vi "define.vi"(8 "error in (no error)":errorcluster, 11 "TrajectoryMH100122AODRAPS in":refnum<class "TrajectoryMH100122AODRAPS.lvclass">) -> (0 "error out":errorcluster, 3 "TrajectoryMH100122AODRAPS out":refnum<class "TrajectoryMH100122AODRAPS.lvclass">)   [LabVIEW 2010, in "TrajectoryMH100122AODRAPS.lvclass"]
doc: "modal dialog on which the user can set the trajectory parameters"
uses:
  TrajectoryMH100122AODRAPS.lvclass
  common/xcontrols/XImage/XImage/XImage.xctl
  common/classes/ImageCollection/ImageCollection/ImageCollection.lvclass
  roi_visualization_cluster.ctl
  common/xcontrols/XImage/XImage/ROI_mode_enum.ctl
  TrajectoryMH100122AODRAPS.lvclass/TrajectoryMH100122AODRAPS.ctl
  <vilib>/Utility/miscctls.llb/LVPointTypeDef.ctl
  common/classes/SpaceVector/SpaceVector/SpaceVector.lvclass
  class_data.vi
  common/classes/ErrorController/ErrorController/class_data.vi
  common/classes/ErrorController/ErrorController/ErrorController.lvclass
  common/classes/Box/Box/Box.lvclass
panel:
  in  "button: ok":bool
  in  "button: cancel":bool
  in  "button: reset":bool
  in  "XImage":refnum<class "ImageCollection.lvclass">(xcontrol)
  in  "accept switch":bool=TRUE
  in  "reset switch":bool
  in  "cancel switch":bool=TRUE
  in  "tab":enum32{"User", "ROI points", "About"}(tab)
  out "FOVy":dbl[unit]=0.0003
  out "FOVx":dbl[unit]=0.0003
  in  "enable sub-pattern":bool
  in  "enable ROI numbering":bool caption="enable numbering"
  in  "ROI color":u32(colorbox)=4456192 caption="color"
  in  "extrapolate distance":dbl[unit] min=0.0
  in  "z-step size / frame":u16
  in  "z-offset":u16
  out "# points":i32
  out "# ROIs":i32
  in  "# iteration points":dbl
  in  "winding number":dbl=1.0 min=1.0
  in  "height":dbl=1.0 min=1.0
  in  "diameter":dbl[unit]
  in  "button:plot_3d":bool
  in  "roi table out":T1[](array[typedef]) {"type" items=["point", "line", "poly line", "free line"]}
  # "ROIs"
  # "z-stepping"
  # "TrajectoryAODRAPS"
  # "Developed by Marcel van 't Hoff, University of Zurich, Switzerland"
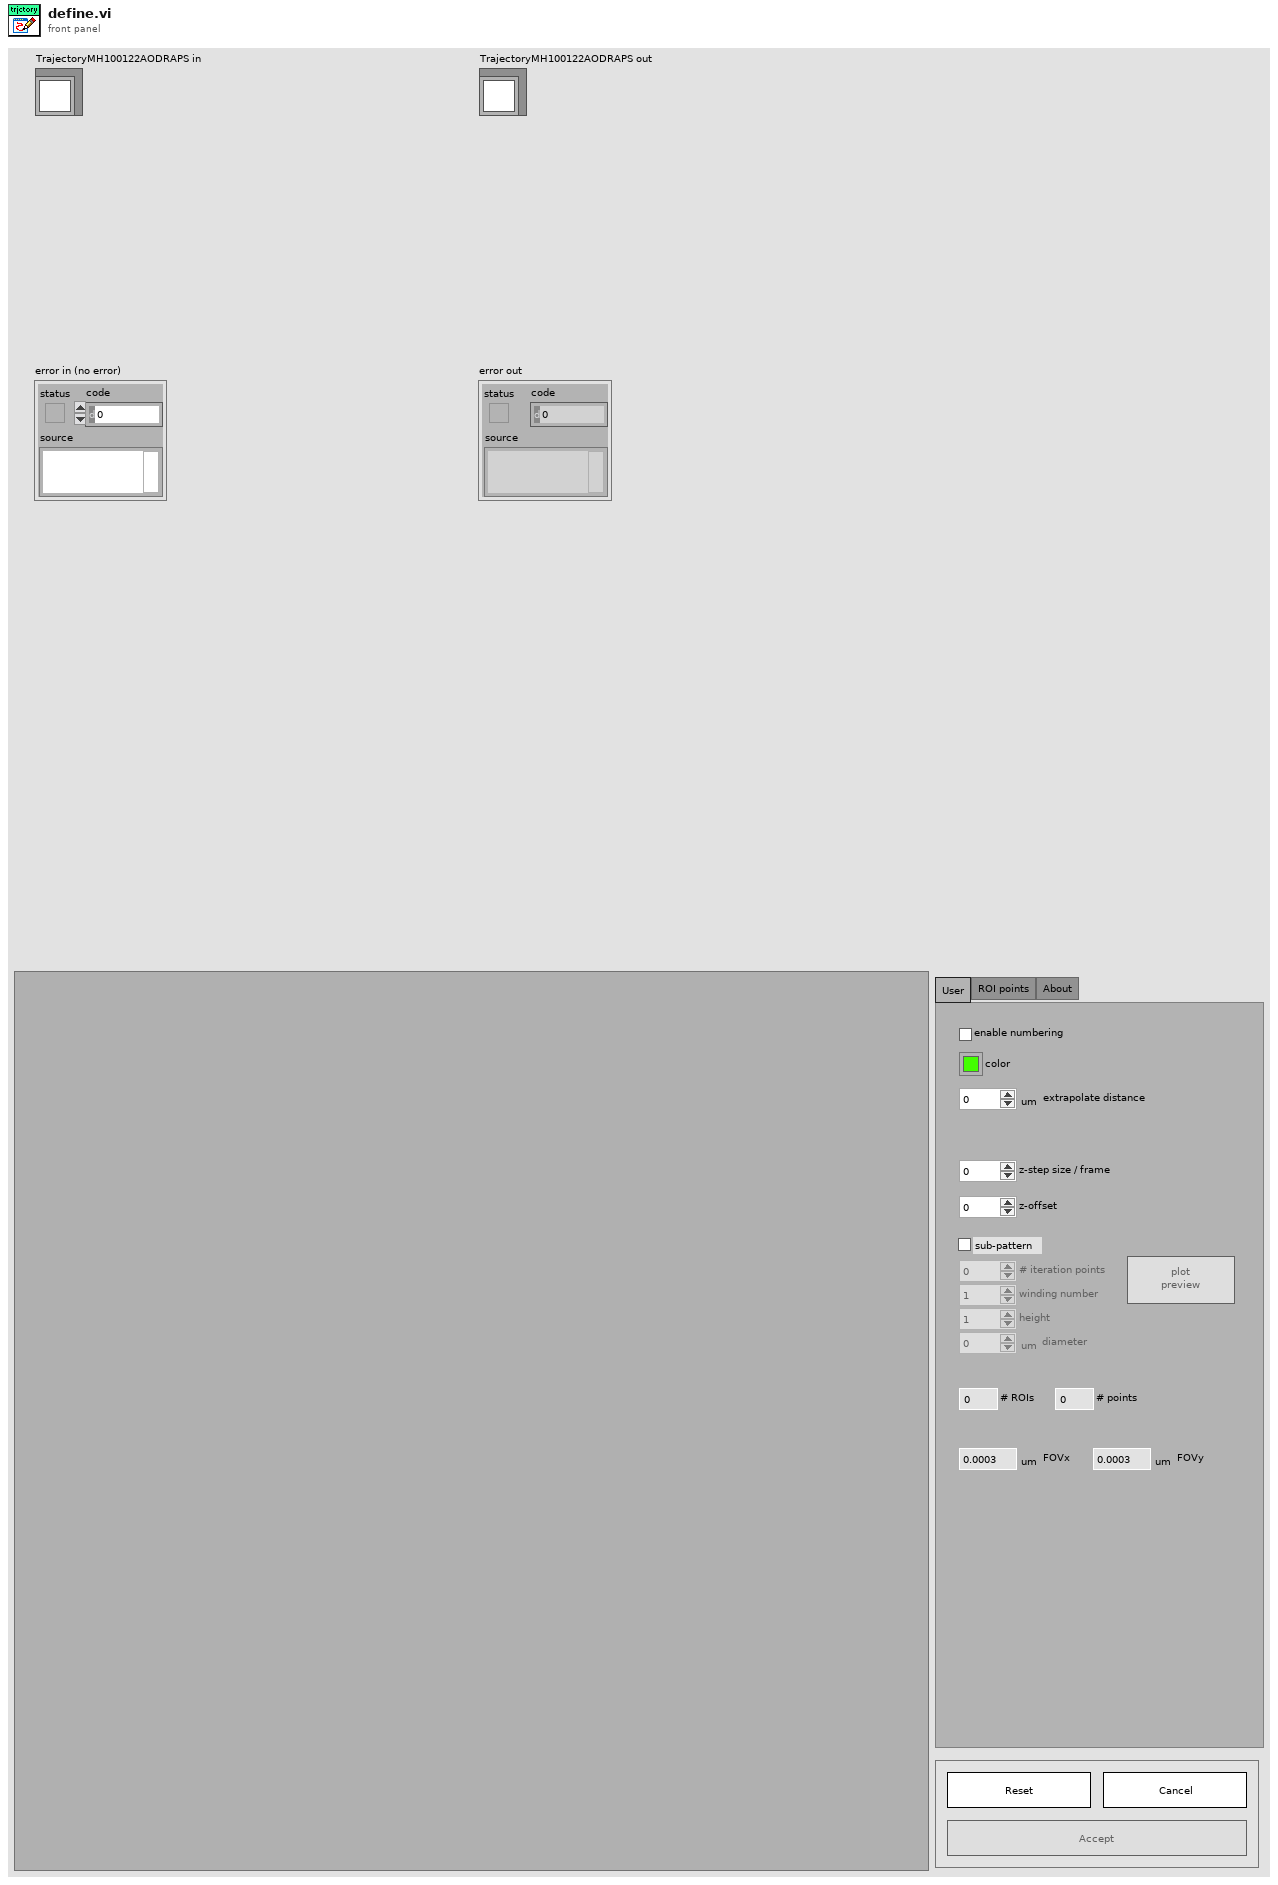
[diagram p1: front panel]
types:
  T1 = typedef "TrajectoryMH100122AODRAPS.lvclass/roi_visualization_cluster.ctl" = cluster{"counter":i32, "type":u16, "activation":enum16{"standard sub-pattern", "long activation"}}
  T2 = typedef "XImage.xctl/ROI_mode_enum.ctl" = enum16{"none", "IMAQROIs", "PointCollection"}
  T3 = typedef "LVPointTypeDef.ctl" = cluster{"Horizontal":i16, "Vertical":i16}
  T4 = cluster{"Global Rectangle":i32[], "Contours":cluster{"Contour Type":u32, "ROI Type":u32, "Points":i32[]}[]}[]
  T5 = enum8{"Enabled", "Disabled", "Disabled and Grayed Out"}
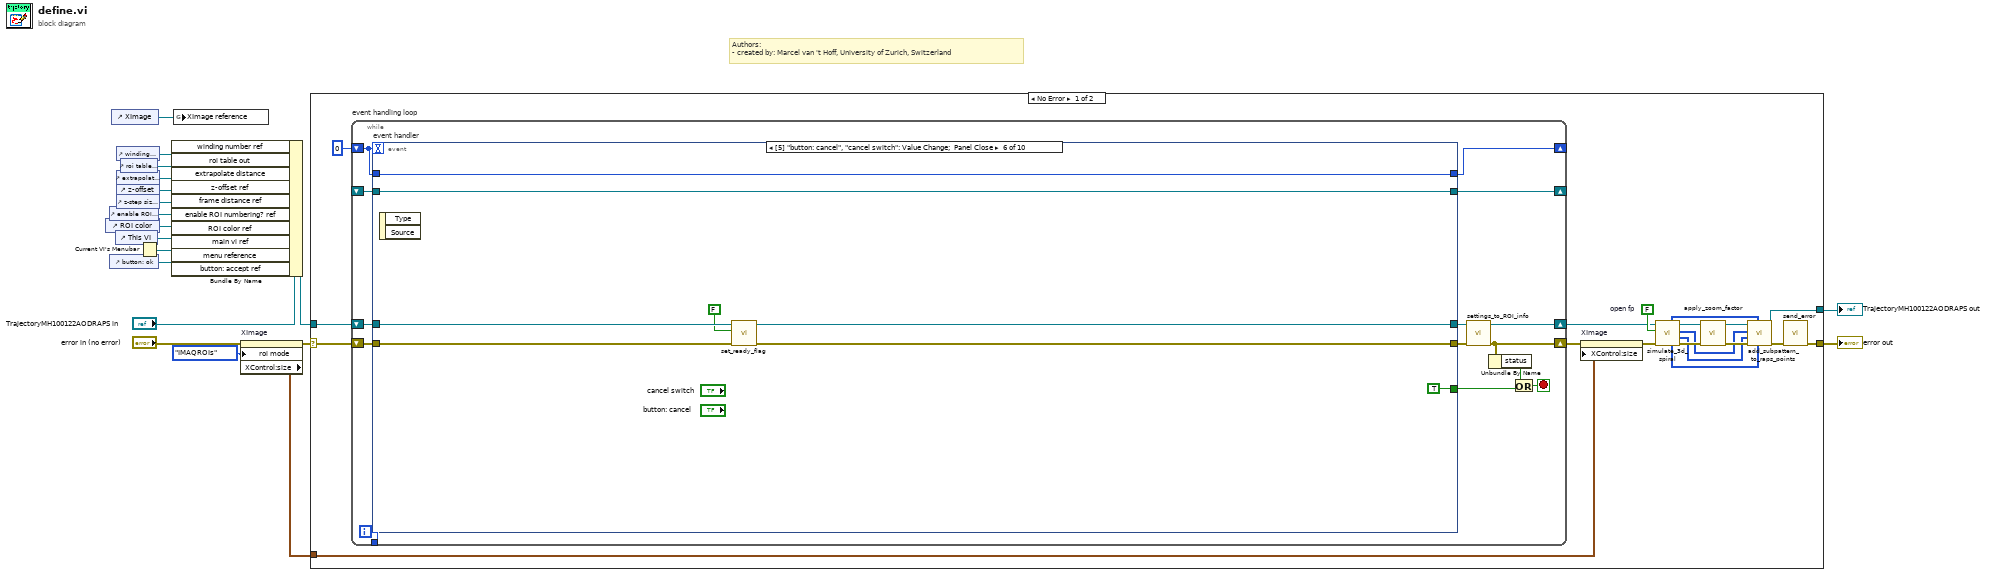
[diagram p0: block diagram]
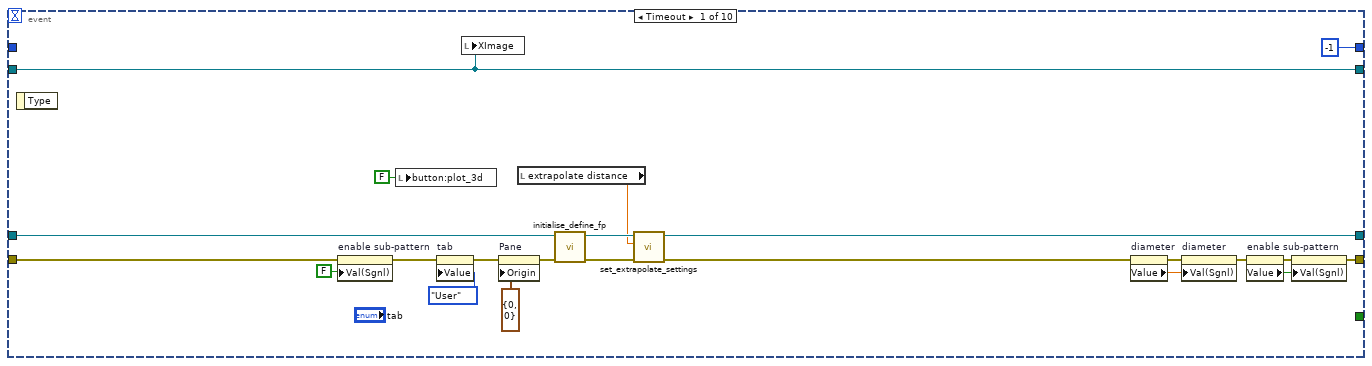
[diagram p2: hidden frame]
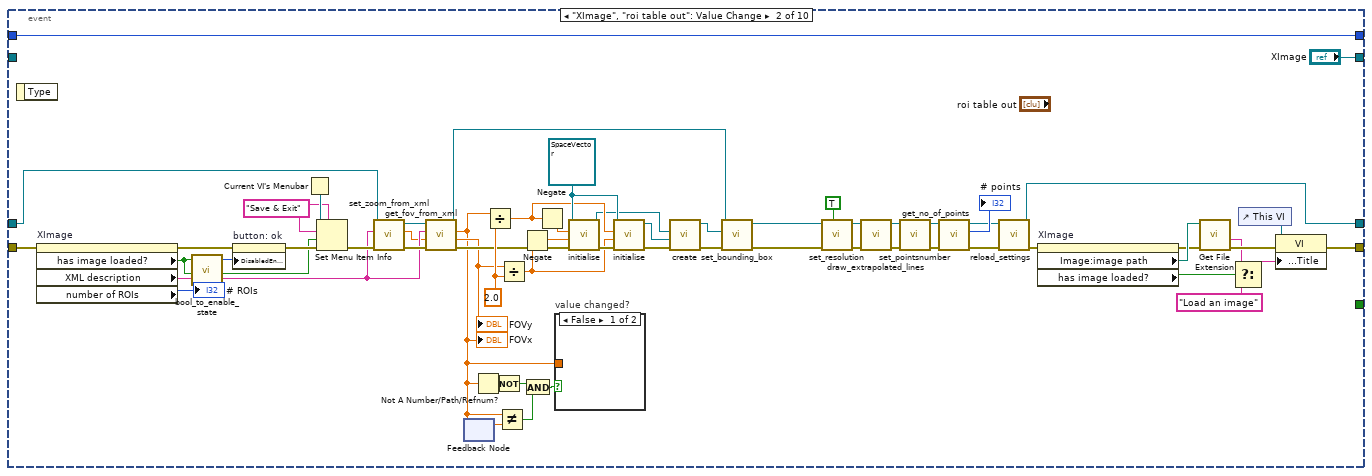
[diagram p3: hidden frame]
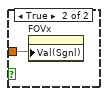
[diagram p4: hidden frame]
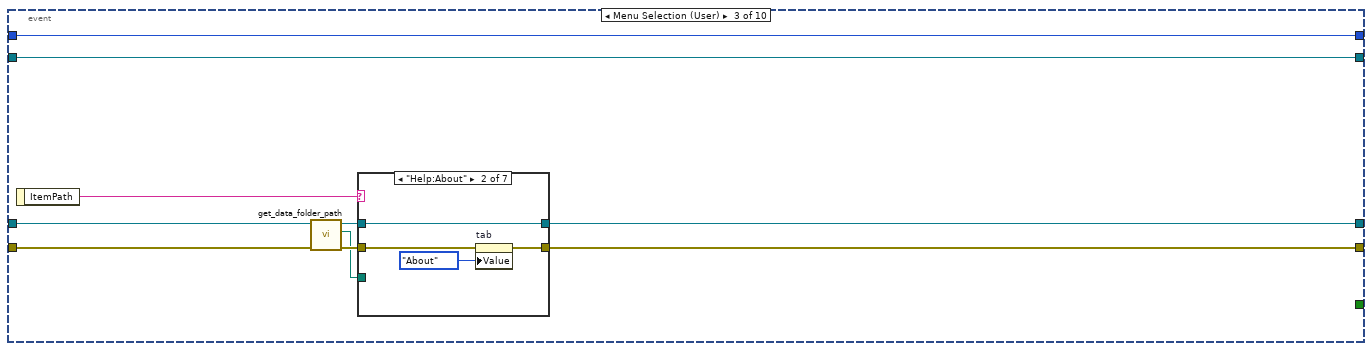
[diagram p5: hidden frame]
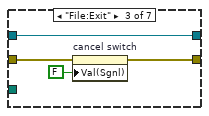
[diagram p7: hidden frame]
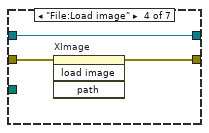
[diagram p8: hidden frame]
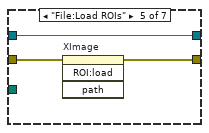
[diagram p9: hidden frame]
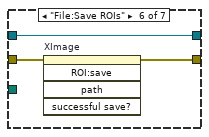
[diagram p10: hidden frame]
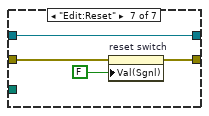
[diagram p11: hidden frame]
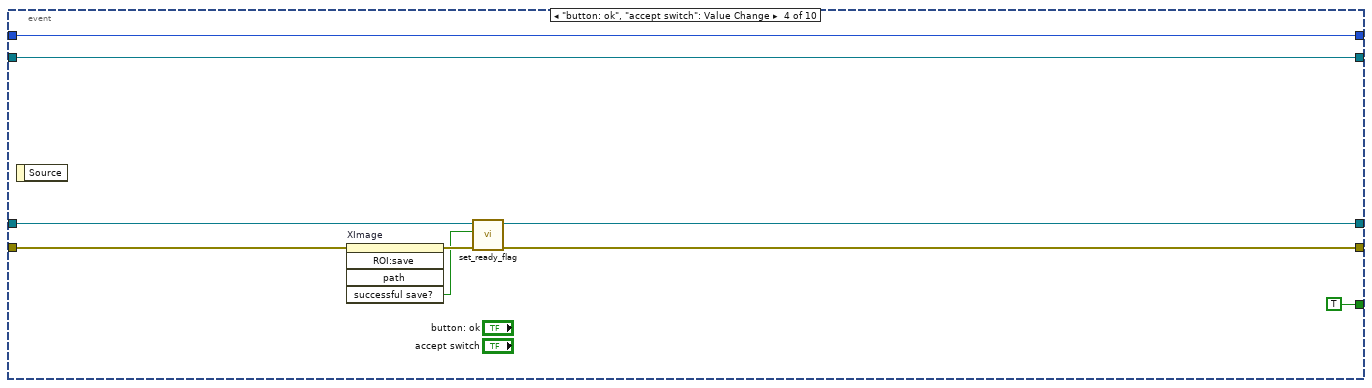
[diagram p12: hidden frame]
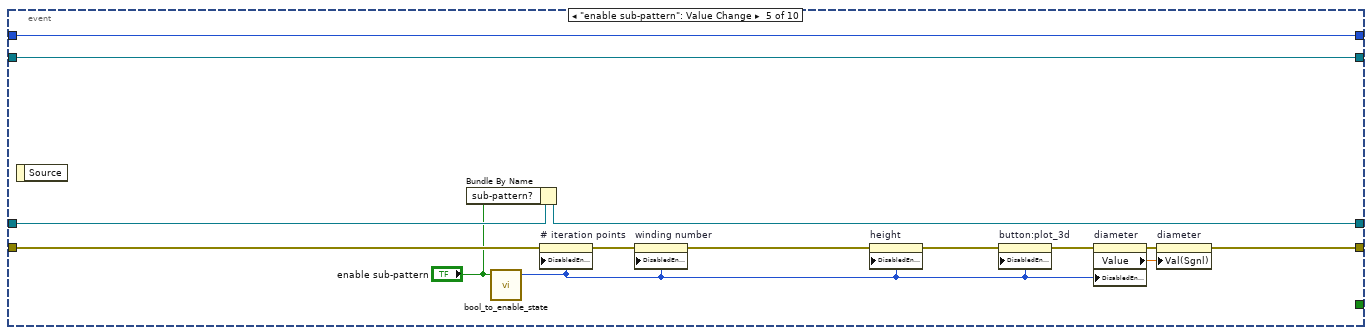
[diagram p13: hidden frame]
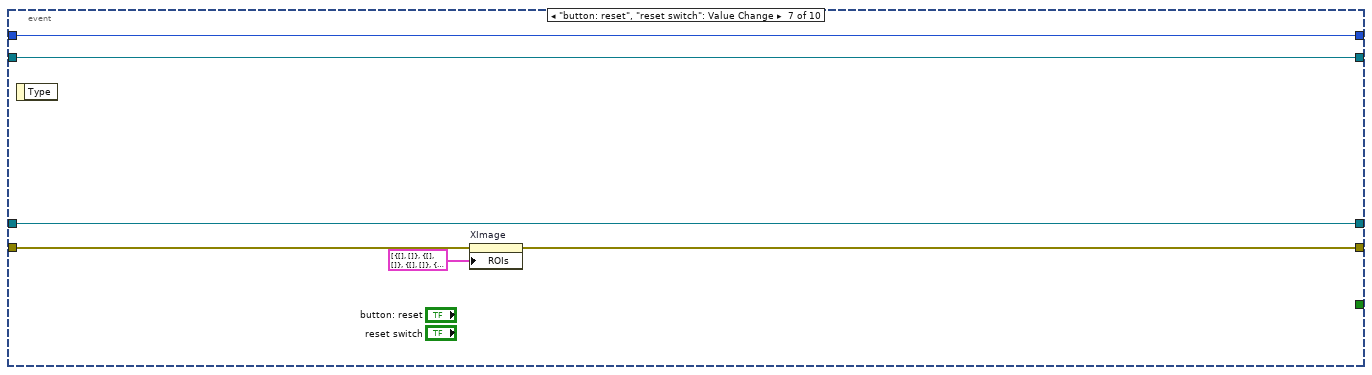
[diagram p14: hidden frame]
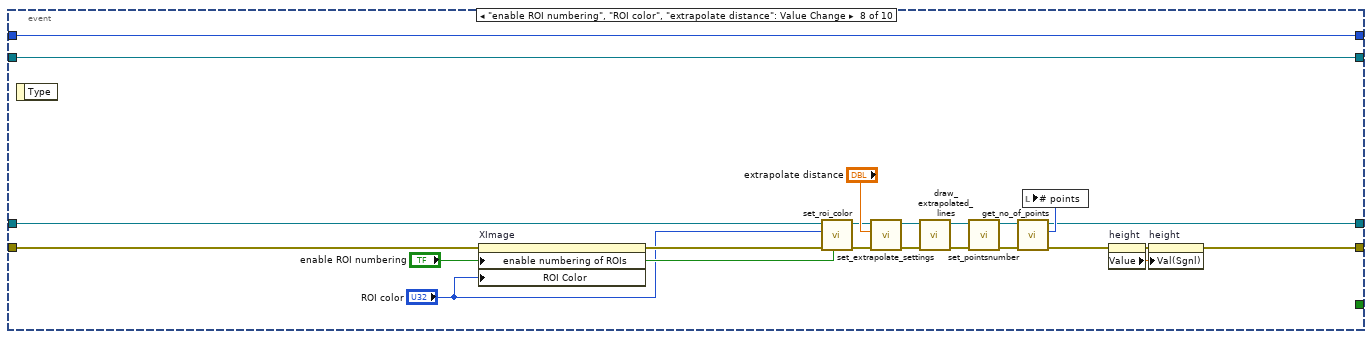
[diagram p15: hidden frame]
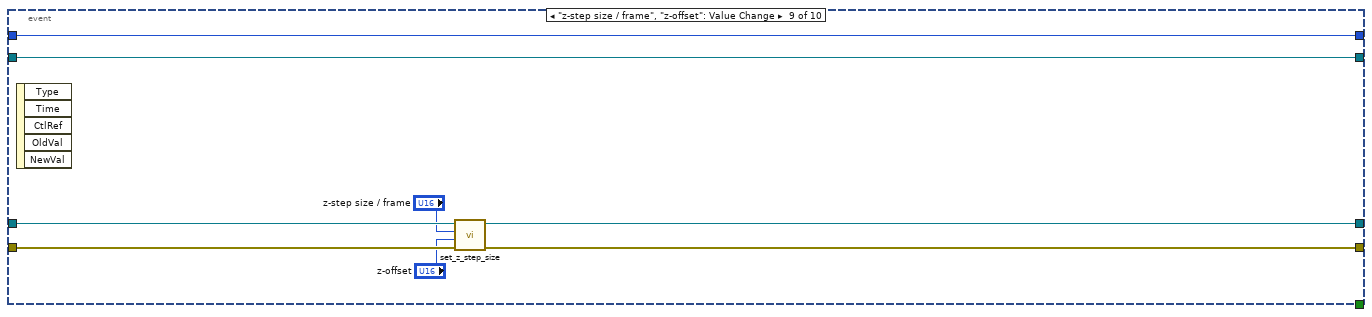
[diagram p16: hidden frame]
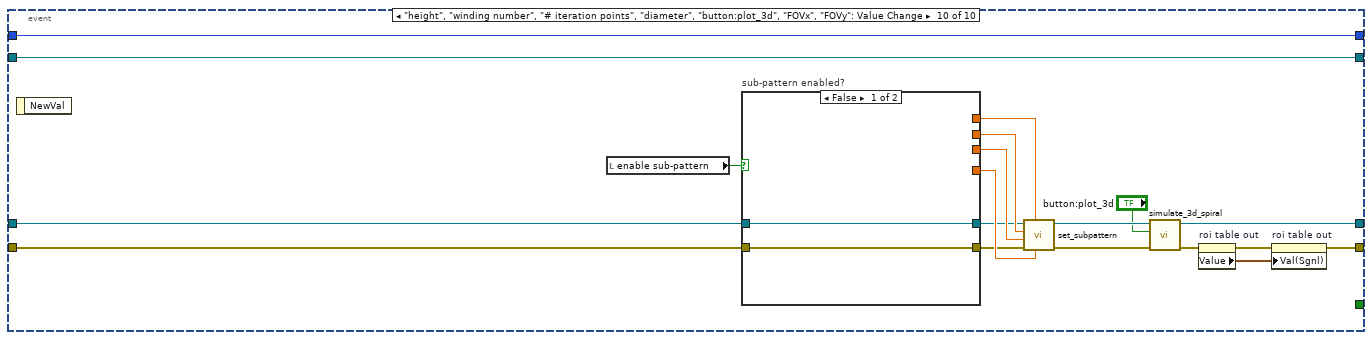
[diagram p17: hidden frame]
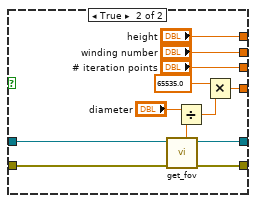
[diagram p18: hidden frame]
diagram:
  # "Authors: \n- created by: Marcel van 't Hoff, University of Zurich, Switzerland"
  n1 = control-ref of="ROI color"() -> (w15:refnum<vi>)
  n2 = control-ref of="enable ROI numbering"() -> (w16:refnum<vi>)
  n3 = control-ref of="button: ok"() -> (w14:refnum<vi>)
  n4 = control-ref of="XImage"() -> (w3:refnum<vi>)
  n5 = control-ref of="This VI"() -> (w12:refnum<vi>)
  n6 = control-ref of="winding number"() -> (w4:refnum<vi>)
  n7 = control-ref of="extrapolate distance"() -> (w8:refnum<vi>)
  n8 = control-ref of="z-offset"() -> (w9:refnum<vi>)
  n9 = control-ref of="z-step size / frame"() -> (w17:refnum<vi>)
  n10 = control-ref of="roi table out"() -> (w5:refnum<vi>)
  n11 = Current VI's Menubar() -> (w13:refnum<k9>)
  n12 = Bundle By Name(cluster="TrajectoryMH100122AODRAPS in", "winding number ref"=w4, "roi table out"=w5, "extrapolate distance"=w8, "z-offset ref"=w9, "frame distance ref"=w17, "enable ROI numbering? ref"=w16, "ROI color ref"=w15, "main vi ref"=w12, "menu reference"=w13, "button: accept ref"=w14) -> (w10:refnum<class "TrajectoryMH100122AODRAPS.lvclass">)
  n13 = global write "class_data.vi" "XImage reference"(w3) -> ()
  n14 = property on="XImage" class="XImage (strict)"(error in="error in (no error)", "roi mode"=ROI_mode_enum."IMAQROIs" ("ROI:mode")) -> (error out=w6:errorcluster, "XControl:size"=w1:cluster{"Width":u32, "Height":u32})  [unwired: 1 in, 1 out]
  n15 = case shown="No Error" w6 {
    selector: w6 -> [w38 w270]
    tunnel: [w35 w270] -> w19
    tunnel: [w24 w269] -> w18
    tunnel: w10 -> [w37 w269]
    tunnel: w1 -> [w33 _]
    frame No Error {
      w32 = FALSE  # open fp
      n16 = while "event handling loop" {
        shift-right: [w43] -> w34
        shift-left: w38 -> [w52]
        shift-right: [w41] -> w30
        shift-left: w37 -> [w49]
        shift-right: [w50] -> _
        shift-left: 0 -> [w51]
        shift-right: [w45] -> _
        shift-left: _ -> [w44]
        tunnel: [w39] -> _
        i -> [w39]
        stop <- w47 stop-if-true
        n17 = event "event handler" shown="[5] \"button: cancel\", \"cancel switch\": Value Change;  Panel Close" {
          selector: _ -> [_ _ _ _ _ _ _ _ _ _]
          dyn-events: _ -> [_ _ _ _ _ _ _ _ _ _]
          timeout: w51 -> [_ _ _ _ _ _ _ _ _ _]
          tunnel: [w55 w111 w143 w175 w178 w197 w203 w206 w232 w240] -> w42
          tunnel: w52 -> [w63 w98 w139 w174 w187 w198 w204 w219 w233 w237]
          tunnel: w51 -> [_ w134 w145 w177 w191 w199 w205 w227 w235 w254]
          tunnel: [-1 w134 w145 w177 w191 w199 w205 w227 w235 w254] -> w50
          tunnel: w49 -> [w66 w99 w141 w176 w185 w196 w202 w225 w231 w236]
          tunnel: [w54 w114 w142 w169 w184 w195 w202 w210 w229 w244] -> w40
          tunnel: [_ _ _ TRUE ("x .or. y?") _ TRUE ("x .or. y?") _ _ _ _] -> w46
          tunnel: [w71 "XImage" w136 w170 w190 w192 w200 w226 w234 w253] -> w45
          tunnel: w44 -> [w71 _ w136 w170 w190 w192 w200 w226 w234 w253]
          event Timeout {
            n18 = event-data() -> ()  [unwired: 1 in, 1 out]
            n19 = property on="enable sub-pattern" class="Bool (strict)"(error in=w63, "Val(Sgnl)"=FALSE ("Value (Signaling)")) -> (error out=w62:errorcluster)  [unwired: 1 in, 1 out]
            n20 = local write "button:plot_3d"(FALSE ("button:plot_3d")) -> ()
            n21 = property on="tab" class="TabCtl (strict)"(error in=w62, "Value"=enum32{"User", "ROI points", "About"}."User" ("tab")) -> (error out=w67:errorcluster)  [unwired: 1 in, 1 out]
            n22 = local write "XImage"(w71) -> ()
            n23 = property on="Pane" class="Pane"(error in=w67, "Origin"=T3 {"Horizontal"=0, "Vertical"=0}) -> (error out=w72:errorcluster)  [unwired: 1 in, 1 out]
            n24 = local read "extrapolate distance"() -> (w68:dbl[unit])
            n25 = call-dynamic "initialise_define_fp.vi"("error in (no error)"=w72, "TrajectoryMH100122AODRAPS in"=w66) -> ("error out"=w69:errorcluster, "TrajectoryMH100122AODRAPS out"=w70:refnum<class "TrajectoryMH100122AODRAPS.lvclass">)  [unwired: 8 in]
            n26 = call-dynamic "set_extrapolate_settings.vi"("error in (no error)"=w69, "extrapolate distance"=w68, "TrajectoryMH100122AODRAPS in"=w70) -> ("error out"=w53:errorcluster, "TrajectoryMH100122AODRAPS out"=w54:refnum<class "TrajectoryMH100122AODRAPS.lvclass">)  [unwired: 7 in]
            n27 = property on="diameter" class="DigNum (strict)"(error in=w53) -> (error out=w59:errorcluster, "Value"=w60:dbl[unit])  [unwired: 1 in, 1 out]
            n28 = property on="diameter" class="DigNum (strict)"(error in=w59, "Val(Sgnl)"=w60) -> (error out=w56:errorcluster)  [unwired: 1 in, 1 out]
            n29 = property on="enable sub-pattern" class="Bool (strict)"(error in=w56) -> (error out=w57:errorcluster, "Value"=w58:bool)  [unwired: 1 in, 1 out]
            n30 = property on="enable sub-pattern" class="Bool (strict)"(error in=w57, "Val(Sgnl)"=w58) -> (error out=w55:errorcluster)  [unwired: 1 in, 1 out]
          }
          event "XImage", "roi table out": Value Change {
            w96 = refnum<class "SpaceVector.lvclass"> refnum ("SpaceVector in")
            w97 = 2.0
            w126 = "Save & Exit" ("item tag")
            n31 = event-data() -> ()  [unwired: 1 in, 1 out]
            n32 = property on="XImage" class="XImage (strict)"(error in=w98) -> (error out=w133:errorcluster, "has image loaded?"=w127:bool, "XML description"=w100:string, "number of ROIs"=→"# ROIs":i32)  [unwired: 1 in, 1 out]
            n33 = call "bool_to_enable_state.vi"("boolean in"=w127) -> ("enabled status out"=w132:T5)  [unwired: 4 in]
            n34 = property on="button: ok" class="Bool"(error in=w133, "DisabledEnum"=w132) -> (error out=w129:errorcluster)  [unwired: 1 in, 1 out]
            n35 = Current VI's Menubar() -> (w130:refnum<k9>)
            n36 = Set Menu Item Info(7:w126, 8:w129, 9:w127, 10:w126, 11:w130) -> (0:w128:errorcluster)  [unwired: 2 in, 1 out]
            n37 = call-dynamic "set_zoom_from_xml.vi"("error in (no error)"=w128, "XML string"=w100, "TrajectoryMH100122AODRAPS in"=w99) -> ("error out"=w101:errorcluster, "zoom"=w77:dbl, "TrajectoryMH100122AODRAPS out"=w102:refnum<class "TrajectoryMH100122AODRAPS.lvclass">)  [unwired: 6 in]
            n38 = call-dynamic "get_fov_from_xml.vi"("error in (no error)"=w101, "zoom"=w77, "XML string"=w100, "TrajectoryMH100122AODRAPS in"=w102) -> ("error out"=w85:errorcluster, "FOVy"=w76:dbl[unit], "FOVx"=w75:dbl[unit], "TrajectoryMH100122AODRAPS out"=w84:refnum<class "TrajectoryMH100122AODRAPS.lvclass">)  [unwired: 4 in]
            "FOVy" <- w76
            "FOVx" <- w75
            n39 = feedback-in #1(w75) -> ()
            n40 = feedback #1() -> (w103:dbl[unit])  [unwired: 1 in]
            n41 = Not A Number/Path/Refnum?(number/path/refnum=w75) -> (NaN/Path/Refnum?=w81:bool)
            n42 = Divide(x=w75, y=w97) -> (x/y=w94:dbl[unit])
            n43 = Not(x=w81) -> (.not. x?=w80:bool)
            n44 = Not Equal?(x=w75, y=w103) -> (x != y?=w79:bool)
            n45 = Divide(x=w76, y=w97) -> (x/y=w93:dbl[unit])
            n46 = Negate(x=w93) -> (-x=w89:dbl[unit])
            n47 = And(x=w80, y=w79) -> (x .and. y?=w78:bool)
            n48 = Negate(x=w94) -> (-x=w90:dbl[unit])
            n49 = case "value changed?" shown="False" w78 {
              tunnel: w75 -> [_ w135]
              frame False {
              }
              frame True {
                n50 = property on="FOVx" class="DigNum (strict)"("Val(Sgnl)"=w135) -> ()  [unwired: 2 in, 2 out]
              }
            }
            n51 = call "initialise.vi"("error in (no error)"=w85, "y"=w89, "x"=w90, "SpaceVector in"=w96) -> ("error out"=w95:errorcluster, "SpaceVector out"=w88:refnum<class "SpaceVector.lvclass">)  [unwired: 6 in]
            n52 = call "initialise.vi"("error in (no error)"=w95, "y"=w93, "x"=w94, "SpaceVector in"=w96) -> ("error out"=w92:errorcluster, "SpaceVector out"=w87:refnum<class "SpaceVector.lvclass">)  [unwired: 6 in]
            n53 = call "create.vi"("error in (no error)"=w92, "maximum"=w87, "minimum"=w88) -> ("error out"=w91:errorcluster, "Box out"=w86:refnum<class "Box.lvclass">)  [unwired: 7 in]
            n54 = call-dynamic "set_bounding_box.vi"("error in (no error)"=w91, "Box.lvclass"=w86, "GenericTrajectory in"=w84) -> ("error out"=w83:errorcluster, "GenericTrajectory out"=w82:refnum<class "TrajectoryMH100122AODRAPS.lvclass">)  [unwired: 7 in]
            n55 = call-dynamic "set_resolution.vi"("get from XImage (F)"=TRUE, "error in (no error)"=w83, "TrajectoryMH100122AODRAPS in"=w82) -> ("error out"=w122:errorcluster, "TrajectoryMH100122AODRAPS out"=w123:refnum<class "TrajectoryMH100122AODRAPS.lvclass">)  [unwired: 7 in]
            n56 = call-dynamic "draw_extrapolated_lines.vi"("error in (no error)"=w122, "TrajectoryMH100122AODRAPS in"=w123) -> ("error out"=w118:errorcluster, "TrajectoryMH100122AODRAPS out"=w120:refnum<class "TrajectoryMH100122AODRAPS.lvclass">)  [unwired: 8 in]
            n57 = call-dynamic "set_pointsnumber.vi"("error in (no error)"=w118, "TrajectoryMH100122AODRAPS in"=w120) -> ("error out"=w121:errorcluster, "TrajectoryMH100122AODRAPS out"=w119:refnum<class "TrajectoryMH100122AODRAPS.lvclass">)  [unwired: 8 in]
            n58 = call-dynamic "get_no_of_points.vi"("error in (no error)"=w121, "TrajectoryMH100122AODRAPS in"=w119) -> ("error out"=w115:errorcluster, "no. of points"=→"# points":i32, "TrajectoryMH100122AODRAPS out"=w116:refnum<class "TrajectoryMH100122AODRAPS.lvclass">)  [unwired: 7 in]
            n59 = call-dynamic "reload_settings.vi"("error in (no error)"=w115, "TrajectoryMH100122AODRAPS in"=w116) -> ("error out"=w109:errorcluster, "TrajectoryMH100122AODRAPS out"=w114:refnum<class "TrajectoryMH100122AODRAPS.lvclass">)  [unwired: 8 in]
            n60 = property on="XImage" class="XImage (strict)"(error in=w109) -> (error out=w108:errorcluster, "Image:image path"=w110:path, "has image loaded?"=w107:bool)  [unwired: 1 in, 1 out]
            n61 = call <vilib>:"Get File Extension.vi"("error in (no error)"=w108, "file"=w110) -> ("error out"=w112:errorcluster, "filename without extension"=w106:string)  [unwired: 6 in, 2 out]
            n62 = Select(t=w106, s=w107, f="Load an image") -> (s? t:f=w105:string)
            n63 = control-ref of="This VI"() -> (w113:refnum<vi>)
            n64 = property class="VI"(reference=w113, error in=w112, "Front Panel.Title"=w105) -> (error out=w111:errorcluster)  [unwired: 1 out]
          }
          event Menu Selection (User) {
            n65 = event-data() -> ("ItemPath"=w144:string)  [unwired: 1 in]
            n66 = call-dynamic "get_data_folder_path.vi"("error in (no error)"=w139, "GenericComponent in"=w141) -> ("error out"=w138:errorcluster, "data folder path"=w137:path, "GenericComponent out"=w140:refnum<class "TrajectoryMH100122AODRAPS.lvclass">)  [unwired: 7 in]
            n67 = case shown="\"Help:About\"" w144 {
              tunnel: w138 -> [w147 w150 w154 w157 w160 w163 w167]
              tunnel: [w147 w149 w153 w156 w159 w162 w166] -> w143
              tunnel: [w146 w151 w155 w158 w161 w164 w168] -> w142
              tunnel: w140 -> [w146 w151 w155 w158 w161 w164 w168]
              tunnel: w137 -> [_ _ _ _ _ _ _]
              frame Default {
              }
              frame "Help:About" {
                n68 = property on="tab" class="TabCtl (strict)"(error in=w150, "Value"=enum32{"User", "ROI points", "About"}."About" ("tab")) -> (error out=w149:errorcluster)  [unwired: 1 in, 1 out]
              }
              frame "File:Exit" {
                n69 = property on="cancel switch" class="Bool (strict)"(error in=w154, "Val(Sgnl)"=FALSE ("Value (Signaling)")) -> (error out=w153:errorcluster)  [unwired: 1 in, 1 out]
              }
              frame "File:Load image" {
                n70 = invoke on="XImage" class="XImage (strict)" method="load image"(error in=w157) -> (error out=w156:errorcluster)  [unwired: 3 in, 3 out]
              }
              frame "File:Load ROIs" {
                n71 = invoke on="XImage" class="XImage (strict)" method="ROI:load"(error in=w160) -> (error out=w159:errorcluster)  [unwired: 3 in, 3 out]
              }
              frame "File:Save ROIs" {
                n72 = invoke on="XImage" class="XImage (strict)" method="ROI:save"(error in=w163) -> (error out=w162:errorcluster)  [unwired: 4 in, 4 out]
              }
              frame "Edit:Reset" {
                n73 = property on="reset switch" class="Bool (strict)"(error in=w167, "Val(Sgnl)"=FALSE ("Value (Signaling)")) -> (error out=w166:errorcluster)  [unwired: 1 in, 1 out]
              }
            }
          }
          event "button: ok", "accept switch": Value Change {
            n74 = event-data() -> ()  [unwired: 1 in, 1 out]
            n75 = invoke on="XImage" class="XImage (strict)" method="ROI:save"(error in=w174) -> (error out=w173:errorcluster, "successful save?"=w171:bool)  [unwired: 4 in, 3 out]
            n76 = call-dynamic "set_ready_flag.vi"("error in (no error)"=w173, "ready for initialisation?"=w171, "GenericTrajectory in"=w176) -> ("error out"=w175:errorcluster, "GenericTrajectory out"=w169:refnum<class "TrajectoryMH100122AODRAPS.lvclass">)  [unwired: 7 in]
          }
          event "enable sub-pattern": Value Change {
            n77 = event-data() -> ()  [unwired: 1 in, 1 out]
            n78 = Bundle By Name(cluster=w185, "sub-pattern?"="enable sub-pattern") -> (w184:refnum<class "TrajectoryMH100122AODRAPS.lvclass">)
            n79 = call "bool_to_enable_state.vi"("boolean in"="enable sub-pattern") -> ("enabled status out"=w186:T5)  [unwired: 4 in]
            n80 = property on="# iteration points" class="DigNum (strict)"(error in=w187, "DisabledEnum"=w186) -> (error out=w189:errorcluster)  [unwired: 1 in, 1 out]
            n81 = property on="winding number" class="DigNum (strict)"(error in=w189, "DisabledEnum"=w186) -> (error out=w188:errorcluster)  [unwired: 1 in, 1 out]
            n82 = property on="height" class="DigNum (strict)"(error in=w188, "DisabledEnum"=w186) -> (error out=w182:errorcluster)  [unwired: 1 in, 1 out]
            n83 = property on="button:plot_3d" class="Bool (strict)"(error in=w182, "DisabledEnum"=w186) -> (error out=w181:errorcluster)  [unwired: 1 in, 1 out]
            n84 = property on="diameter" class="DigNum (strict)"(error in=w181, "DisabledEnum"=w186) -> (error out=w179:errorcluster, "Value"=w180:dbl[unit])  [unwired: 1 in, 1 out]
            n85 = property on="diameter" class="DigNum (strict)"(error in=w179, "Val(Sgnl)"=w180) -> (error out=w178:errorcluster)  [unwired: 1 in, 1 out]
          }
          event "button: cancel", "cancel switch": Value Change; Panel Close {
            n86 = event-data() -> ()  [unwired: 1 in, 2 out]
            n87 = call-dynamic "set_ready_flag.vi"("error in (no error)"=w198, "ready for initialisation?"=FALSE, "GenericTrajectory in"=w196) -> ("error out"=w197:errorcluster, "GenericTrajectory out"=w195:refnum<class "TrajectoryMH100122AODRAPS.lvclass">)  [unwired: 7 in]
          }
          event "button: reset", "reset switch": Value Change {
            n88 = event-data() -> ()  [unwired: 1 in, 1 out]
            n89 = property on="XImage" class="XImage (strict)"(error in=w204, "ROIs"=T4 [{"Global Rectangle"=[], "Contours"=[]}, {"Global Rectangle"=[], "Contours"=[]}, {"Global Rectangle"=[], "Contours"=[]}, {"Global Rectangle"=[], "Contours"=[]}, {"Global Rectangle"=[], "Contours"=[]}, {"Global Rectangle"=[], "Contours"=[]}, {"Global Rectangle"=[], "Contours"=[]}, {"Global Rectangle"=[], "Contours"=[]}, {"Global Rectangle"=[], "Contours"=[]}, {"Global Rectangle"=[], "Contours"=[]}] ("ROI:ROIs")) -> (error out=w203:errorcluster)  [unwired: 1 in, 1 out]
          }
          event "enable ROI numbering", "ROI color", "extrapolate distance": Value Change {
            n90 = event-data() -> ()  [unwired: 1 in, 1 out]
            n91 = property on="XImage" class="XImage (strict)"(error in=w219, "enable numbering of ROIs"="enable ROI numbering", "ROI Color"="ROI color") -> (error out=w218:errorcluster)  [unwired: 1 in, 1 out]
            n92 = call-dynamic "set_roi_color.vi"("enable ROI numbering"="enable ROI numbering", "error in (no error)"=w218, "ROI color"="ROI color", "TrajectoryMH100122AODRAPS in"=w225) -> ("error out"=w220:errorcluster, "TrajectoryMH100122AODRAPS out"=w223:refnum<class "TrajectoryMH100122AODRAPS.lvclass">)  [unwired: 6 in]
            n93 = call-dynamic "set_extrapolate_settings.vi"("error in (no error)"=w220, "extrapolate distance"="extrapolate distance", "TrajectoryMH100122AODRAPS in"=w223) -> ("error out"=w221:errorcluster, "TrajectoryMH100122AODRAPS out"=w222:refnum<class "TrajectoryMH100122AODRAPS.lvclass">)  [unwired: 7 in]
            n94 = call-dynamic "draw_extrapolated_lines.vi"("error in (no error)"=w221, "TrajectoryMH100122AODRAPS in"=w222) -> ("error out"=w213:errorcluster, "TrajectoryMH100122AODRAPS out"=w215:refnum<class "TrajectoryMH100122AODRAPS.lvclass">)  [unwired: 8 in]
            n95 = call-dynamic "set_pointsnumber.vi"("error in (no error)"=w213, "TrajectoryMH100122AODRAPS in"=w215) -> ("error out"=w214:errorcluster, "TrajectoryMH100122AODRAPS out"=w217:refnum<class "TrajectoryMH100122AODRAPS.lvclass">)  [unwired: 8 in]
            n96 = call-dynamic "get_no_of_points.vi"("error in (no error)"=w214, "TrajectoryMH100122AODRAPS in"=w217) -> ("error out"=w207:errorcluster, "no. of points"=w216:i32, "TrajectoryMH100122AODRAPS out"=w210:refnum<class "TrajectoryMH100122AODRAPS.lvclass">)  [unwired: 7 in]
            n97 = local write "# points"(w216) -> ()
            n98 = property on="height" class="DigNum (strict)"(error in=w207) -> (error out=w208:errorcluster, "Value"=w209:dbl)  [unwired: 1 in, 1 out]
            n99 = property on="height" class="DigNum (strict)"(error in=w208, "Val(Sgnl)"=w209) -> (error out=w206:errorcluster)  [unwired: 1 in, 1 out]
          }
          event "z-step size / frame", "z-offset": Value Change {
            n100 = event-data() -> ()  [unwired: 1 in, 5 out]
            n101 = call-dynamic "set_z_step_size.vi"("error in (no error)"=w233, "z-offset"="z-offset", "z-step size / frame"="z-step size / frame", "TrajectoryMH100122AODRAPS in"=w231) -> ("error out"=w232:errorcluster, "TrajectoryMH100122AODRAPS out"=w229:refnum<class "TrajectoryMH100122AODRAPS.lvclass">)  [unwired: 6 in]
          }
          event "height", "winding number", "# iteration points", "diameter", "button:plot_3d", "FOVx", "FOVy": Value Change {
            n102 = event-data() -> ()  [unwired: 1 in, 1 out]
            n103 = local read "enable sub-pattern"() -> (w245:bool)
            n104 = case "sub-pattern enabled?" shown="False" w245 {
              tunnel: [_ "height"] -> w252
              tunnel: [_ "# iteration points"] -> w251
              tunnel: [_ "winding number"] -> w250
              tunnel: [_ w260] -> w249
              tunnel: w236 -> [w255 w263]
              tunnel: w237 -> [w256 w257]
              tunnel: [w256 w262] -> w239
              tunnel: [w255 w261] -> w238
              frame False {
              }
              frame True {
                n105 = call-dynamic "get_fov.vi"("error in (no error)"=w257, "TrajectoryMH100122AODRAPS in"=w263) -> ("error out"=w262:errorcluster, "TrajectoryMH100122AODRAPS out"=w261:refnum<class "TrajectoryMH100122AODRAPS.lvclass">, "average"=w259:dbl[unit])  [unwired: 5 in, 2 out]
                n106 = Divide(x="diameter", y=w259) -> (x/y=w264:dbl)
                n107 = Multiply(x=65535.0 ("y"), y=w264) -> (x*y=w260:dbl)
              }
            }
            n108 = call-dynamic "set_subpattern.vi"("diameter"=w249, "height"=w252, "error in (no error)"=w239, "number of iteration points"=w251, "winding number"=w250, "TrajectoryMH100122AODRAPS in"=w238) -> ("error out"=w247:errorcluster, "TrajectoryMH100122AODRAPS out"=w248:refnum<class "TrajectoryMH100122AODRAPS.lvclass">)  [unwired: 4 in]
            n109 = call-dynamic "simulate_3d_spiral.vi"("error in (no error)"=w247, "open fp?"="button:plot_3d", "TrajectoryMH100122AODRAPS in"=w248) -> ("error out"=w241:errorcluster, "TrajectoryMH100122AODRAPS out"=w244:refnum<class "TrajectoryMH100122AODRAPS.lvclass">)  [unwired: 3 in, 4 out]
            n110 = property on="roi table out" class="Arr (strict)"(error in=w241) -> (error out=w242:errorcluster, "Value"=w243:T1[])  [unwired: 1 in, 1 out]
            n111 = property on="roi table out" class="Arr (strict)"(error in=w242, "Val(Sgnl)"=w243) -> (error out=w240:errorcluster)  [unwired: 1 in, 1 out]
          }
        }
        n112 = call-dynamic "settings_to_ROI_info.vi"("error in (no error)"=w42, "TrajectoryMH100122AODRAPS in"=w40) -> ("error out"=w43:errorcluster, "TrajectoryMH100122AODRAPS out"=w41:refnum<class "TrajectoryMH100122AODRAPS.lvclass">)  [unwired: 8 in]
        n113 = Unbundle By Name(w43) -> ("status"=w48:bool)
        n114 = Or(x=w48, y=w46) -> (x .or. y?=w47:bool)
      }
      n115 = property on="XImage" class="XImage (strict)"(error in=w34, "XControl:size"=w33) -> (error out=w31:errorcluster)  [unwired: 1 in, 1 out]
      n116 = call-dynamic "simulate_3d_spiral.vi"("error in (no error)"=w31, "open fp?"=w32, "TrajectoryMH100122AODRAPS in"=w30) -> ("error out"=w29:errorcluster, "subpattern delty y"=w22:i32[], "subpattern delta x"=w23:i32[], "TrajectoryMH100122AODRAPS out"=w28:refnum<class "TrajectoryMH100122AODRAPS.lvclass">, "subpattern delta amp"=w20:i32[], "subpattern delta z"=w21:i32[])  [unwired: 3 in]
      n117 = call-dynamic "apply_zoom_factor.vi"("error in (no error)"=w29, "TrajectoryMH100122AODRAPS in"=w28) -> ("error out"=w27:errorcluster, "TrajectoryMH100122AODRAPS out"=w25:refnum<class "TrajectoryMH100122AODRAPS.lvclass">)  [unwired: 8 in]
      n118 = call "add_subpattern_to_raps_points.vi"("subpattern delty amp"=w20, "subpattern delty z"=w21, "error in (no error)"=w27, "subpattern delty y"=w22, "subpattern delta x"=w23, "TrajectoryMH100122AODRAPS in"=w25) -> ("error out"=w26:errorcluster, "TrajectoryMH100122AODRAPS out"=w24:refnum<class "TrajectoryMH100122AODRAPS.lvclass">)  [unwired: 4 in]
      n119 = call "send_error.vi"("error in (no error)"=w26) -> ("error out"=w35:errorcluster)  [unwired: 10 in]
    }
    frame Error {
    }
  }
  "error out" <- w19
  "TrajectoryMH100122AODRAPS out" <- w18
